vi "SaveExperimentInfo.vi"(10 "Filename":path, 11 "MeasureConfig":T1={"Bead locations"=[{"X"=0, "Y"=0}], "ROI"=0, "Experiment base path"=path "", "Image output subdir"="images", "Output mode"=enum."None", "Traces output subdir"="traces", "QTrk Settings"={"Image width"=150, "Image height"=150, "Number of threads (CPU based)"=-1, "CUDA Device"=200, "COM Background correction factor"=128.0, "ZLUT MinRadius"=32.0, "ZLUT Radial sample density"=2.0, "ZLUT Angular sample density"=5.0, "ZLUT ROI Coverage"=50.0, "QI Iterations"=64, "QI MinRadius"=2.0, "QI Radial sample density"=64.0, "QI Angular sample density"=64.0, "QI ROI Coverage"=2.0, "QI Angular Step \nIteration Factor"=30.0, "XCOR Profile Length"=0, "XCOR Profile Width"=2, "XCOR Iterations"=32, "Gaussian 2D Fit Iterations"=8, "Gaussian 2D Sigma (pixels)"=3.0, "Downsample"=0}, "Tracking Config"={"Number of steps"=150, "ZLUT stepsize (um)"=150.0, "Z correction factor"=-1.0, "Start piezo Z (um)"=200.0, "Pixel size (nm)"=128.0, "2D Localization Type"=enum."Quadrant Interpolation", "Z Command (None)"=enum."Nothing", "Z Piezo scale"=FALSE, "ZLUT Building\nimages per frame"=1, "ZLUT Bias correction planes"=1}, "Experiment Name"="", "Program"={"Commands"=[], "Motor Axis accuracy conditions"={"Magnet Z"=0.0, "Magnet rotation"=0.0, "Camera"={"X"=0.0, "Y"=0.0}, "Piezo XY"={"X"=0.0, "Y"=0.0}, "Piezo Z"=0.0}, "Axis flags"={"Magnet Z"=FALSE, "Magnet rotation"=FALSE, "Camera"={"X"=FALSE, "Y"=FALSE}, "Piezo XY"={"X"=FALSE, "Y"=FALSE}, "Piezo Z"=FALSE}}, "ZLUT"=[], "Camera settings"={"Framerate (Hz)"=60, "Exposure time (us)"=5000, "Image size"={"Width"=1280, "Height"=1024}, "Number of buffers"=30}, "Experiment Script"="", "Max frames in memory"=2, "Save traces as binary"=FALSE, "Pixel Calibration Gain Image"="camera_calib_gain.bin", "Pixel Calibration Offset Image"="camera_calib_gain.bin", "Use pixel calibration images"=FALSE, "Internal camera settings"="", "Trace write interval"=100, "ExperimentComment"=""} {"QTrk Settings"."QI ROI Coverage" format="%_2g"; "QTrk Settings"."QI MinRadius" format="%.2f"; "QTrk Settings"."QI Angular sample density" format="%.3f"; "QTrk Settings"."QI Radial sample density" format="%.2f"; "QTrk Settings"."ZLUT Radial sample density" format="%.2f"; "QTrk Settings"."ZLUT MinRadius" format="%.2f"}) -> ()   [LabVIEW 2011]
uses:
  Typedefs/MeasureConfigType.ctl
  Typedefs/MeasureConfigOutputMode.ctl
  qtrk/QTrkLVBinding/QTrkSettings.ctl
  Typedefs/TrackingConfigType.ctl
  qtrk/QTrkLVBinding/QTrkLocalizationType.ctl
  qtrk/QTrkLVBinding/QTrkZCommandType.ctl
  ExperimentProgram/ExperimentProgramType.ctl
  ExperimentProgram/ExProgCommandType.ctl
  ExperimentProgram/ExProgCommandEnumType.ctl
  Motors/MotorAxisEnum.ctl
  Motors/MotorPosType.ctl
  Typedefs/XYf.ctl
  Motors/MotorPosFlagsType.ctl
  Camera/GenericCameraConfigType.ctl
panel:
  # "(used for commands with string parameters)"
  # "-2: Use all devices\n-1: Use best device"
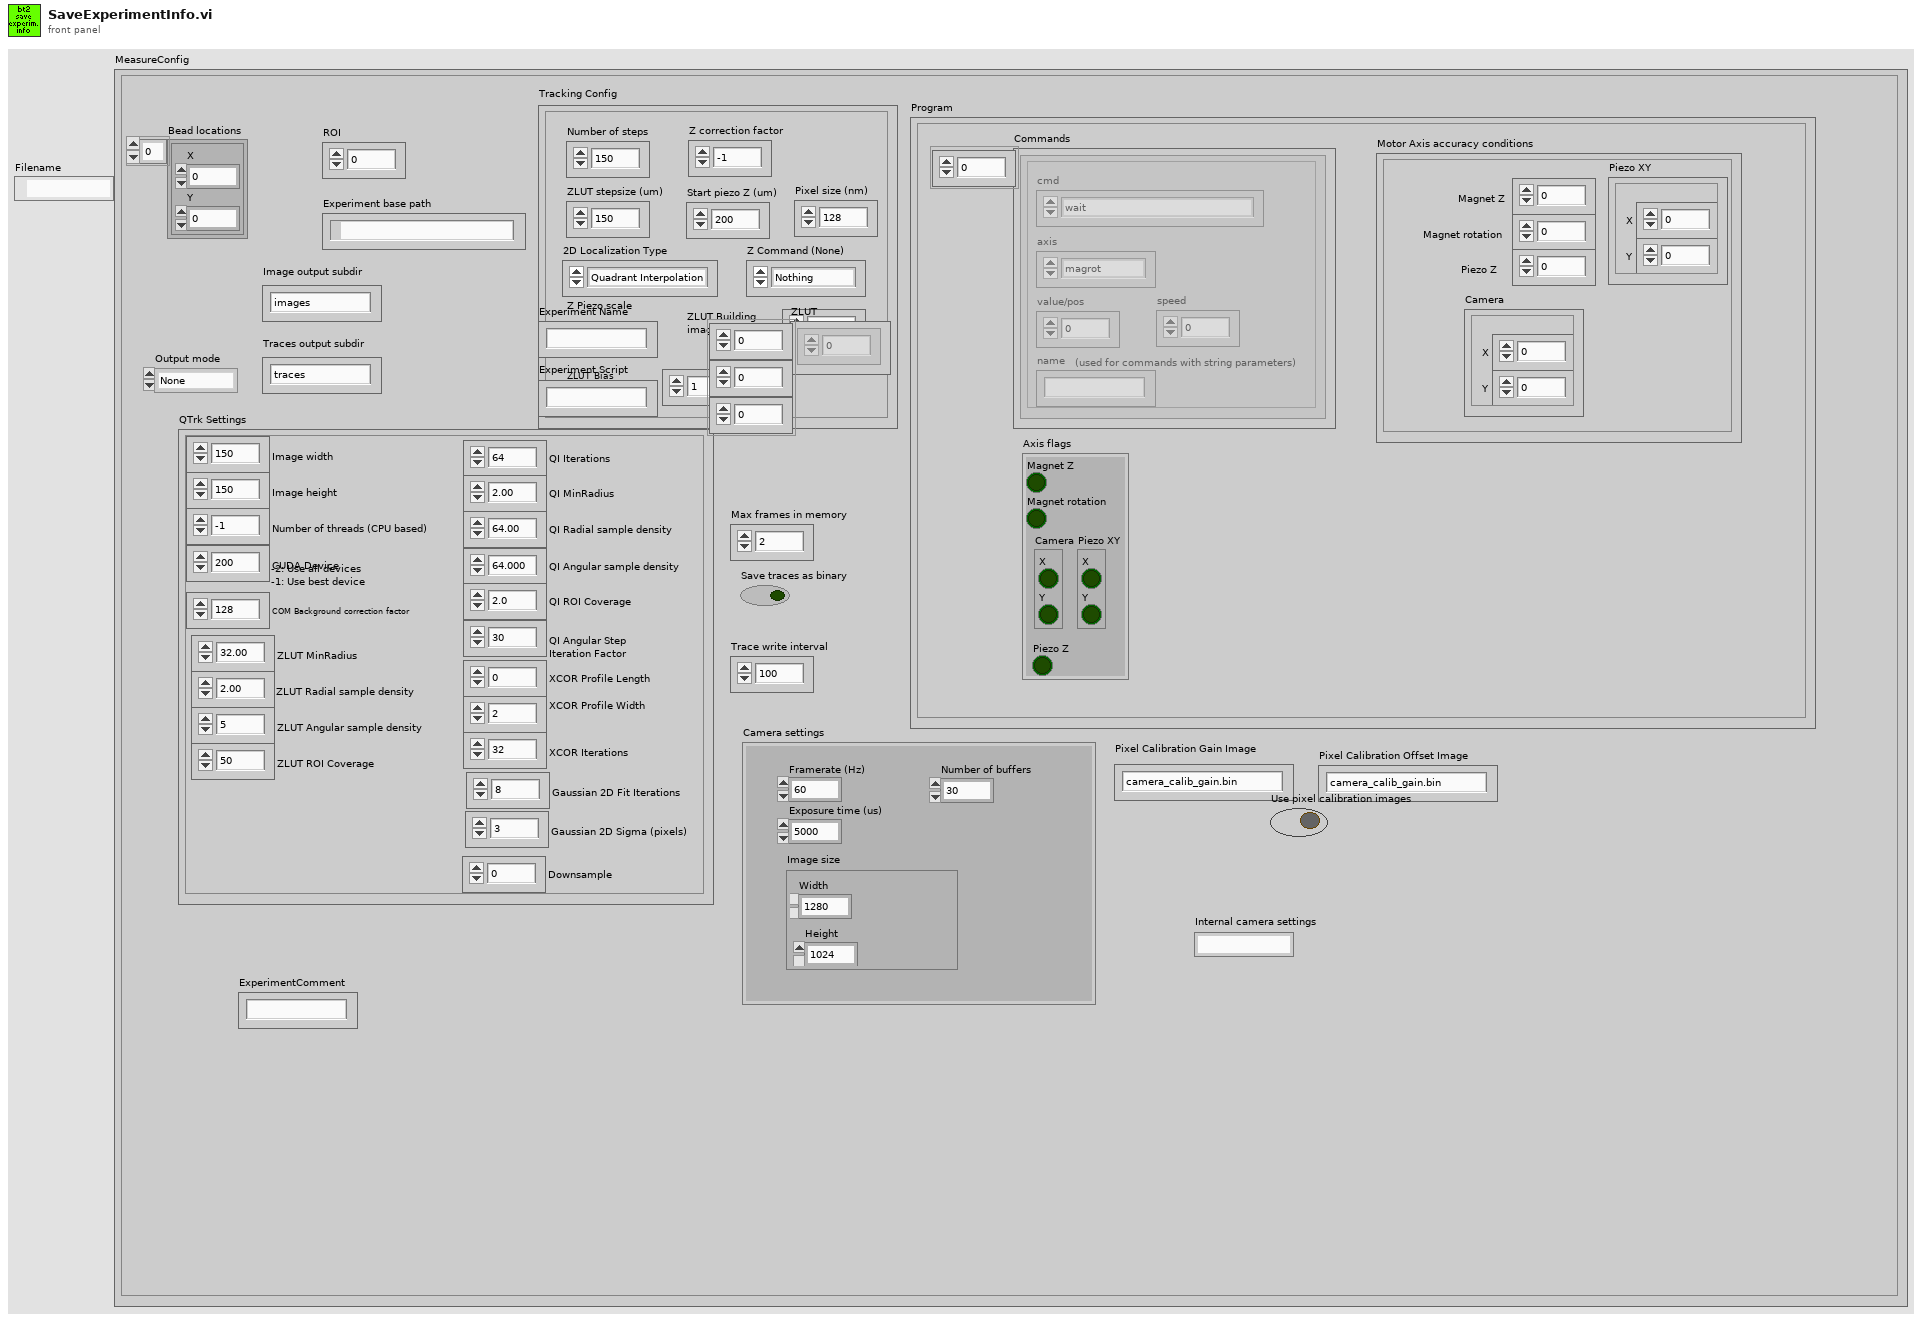
[diagram p1: front panel]
types:
  T1 = typedef "MeasureConfigType.ctl" = cluster{"Bead locations":cluster{"X":i32, "Y":i32}[], "ROI":i32, "Experiment base path":path, "Image output subdir":string, "Output mode":T2, "Traces output subdir":string, "QTrk Settings":T3, "Tracking Config":T4, "Experiment Name":string, "Program":T7, "ZLUT":sgl[][][], "Camera settings":T14, "Experiment Script":string, "Max frames in memory":i32, "Save traces as binary":bool, "Pixel Calibration Gain Image":string, "Pixel Calibration Offset Image":string, "Use pixel calibration images":bool, "Internal camera settings":string, "Trace write interval":i32, "ExperimentComment":string}
  T2 = typedef "MeasureConfigOutputMode.ctl" = enum16{"None", "Track", "SaveImages"}
  T3 = typedef "QTrkSettings.ctl" = cluster{"Image width":i32, "Image height":i32, "Number of threads (CPU based)":i32, "CUDA Device":i32, "COM Background correction factor":sgl, "ZLUT MinRadius":sgl, "ZLUT Radial sample density":sgl, "ZLUT Angular sample density":sgl, "ZLUT ROI Coverage":sgl, "QI Iterations":i32, "QI MinRadius":sgl, "QI Radial sample density":sgl, "QI Angular sample density":sgl, "QI ROI Coverage":sgl, "QI Angular Step \nIteration Factor":sgl, "XCOR Profile Length":i32, "XCOR Profile Width":i32, "XCOR Iterations":i32, "Gaussian 2D Fit Iterations":i32, "Gaussian 2D Sigma (pixels)":sgl, "Downsample":i32}
  T4 = typedef "TrackingConfigType.ctl" = cluster{"Number of steps":i32, "ZLUT stepsize (um)":sgl, "Z correction factor":sgl, "Start piezo Z (um)":sgl, "Pixel size (nm)":sgl, "2D Localization Type":T5, "Z Command (None)":T6, "Z Piezo scale":bool, "ZLUT Building\nimages per frame":i32, "ZLUT Bias correction planes":i32}
  T5 = typedef "QTrkLocalizationType.ctl" = enum16{"Center-of-Mass", "1D Cross-Correlation", "Quadrant Interpolation", "Gaussian 2D MLE", "QI + ZLUTAlign", "ZLUTAlign", "QI + FourierLUT"}
  T6 = typedef "QTrkZCommandType.ctl" = enum16{"Nothing", "ComputeZ", "BuildRadialZLUT", "BuildImageZLUT", "RadialZLUT+ImageZLUT"}
  T7 = typedef "ExperimentProgramType.ctl" = cluster{"Commands":T8[], "Motor Axis accuracy conditions":T11, "Axis flags":T13}
  T8 = typedef "ExProgCommandType.ctl" = cluster{"cmd":T9, "axis":T10, "value/pos":dbl, "speed":dbl, "name":string}
  T9 = typedef "ExProgCommandEnumType.ctl" = enum16{"wait", "move", "event", "idle", "when", "section", "stop"}
  T10 = typedef "MotorAxisEnum.ctl" = enum16{"no axis", "magrot", "magpos", "px", "py", "pz", "camx", "camy"}
  T11 = typedef "MotorPosType.ctl" = cluster{"Magnet Z":dbl, "Magnet rotation":dbl, "Camera":T12, "Piezo XY":T12, "Piezo Z":dbl}
  T12 = typedef "XYf.ctl" = cluster{"X":sgl, "Y":sgl}
  T13 = typedef "MotorPosFlagsType.ctl" = cluster{"Magnet Z":bool, "Magnet rotation":bool, "Camera":cluster{"X":bool, "Y":bool}, "Piezo XY":cluster{"X":bool, "Y":bool}, "Piezo Z":bool}
  T14 = typedef "GenericCameraConfigType.ctl" = cluster{"Framerate (Hz)":i32, "Exposure time (us)":i32, "Image size":cluster{"Width":i32, "Height":i32}, "Number of buffers":i32}
  T15 = enum16{"None", "Normalize", "NormalizeWithoutOffset"}
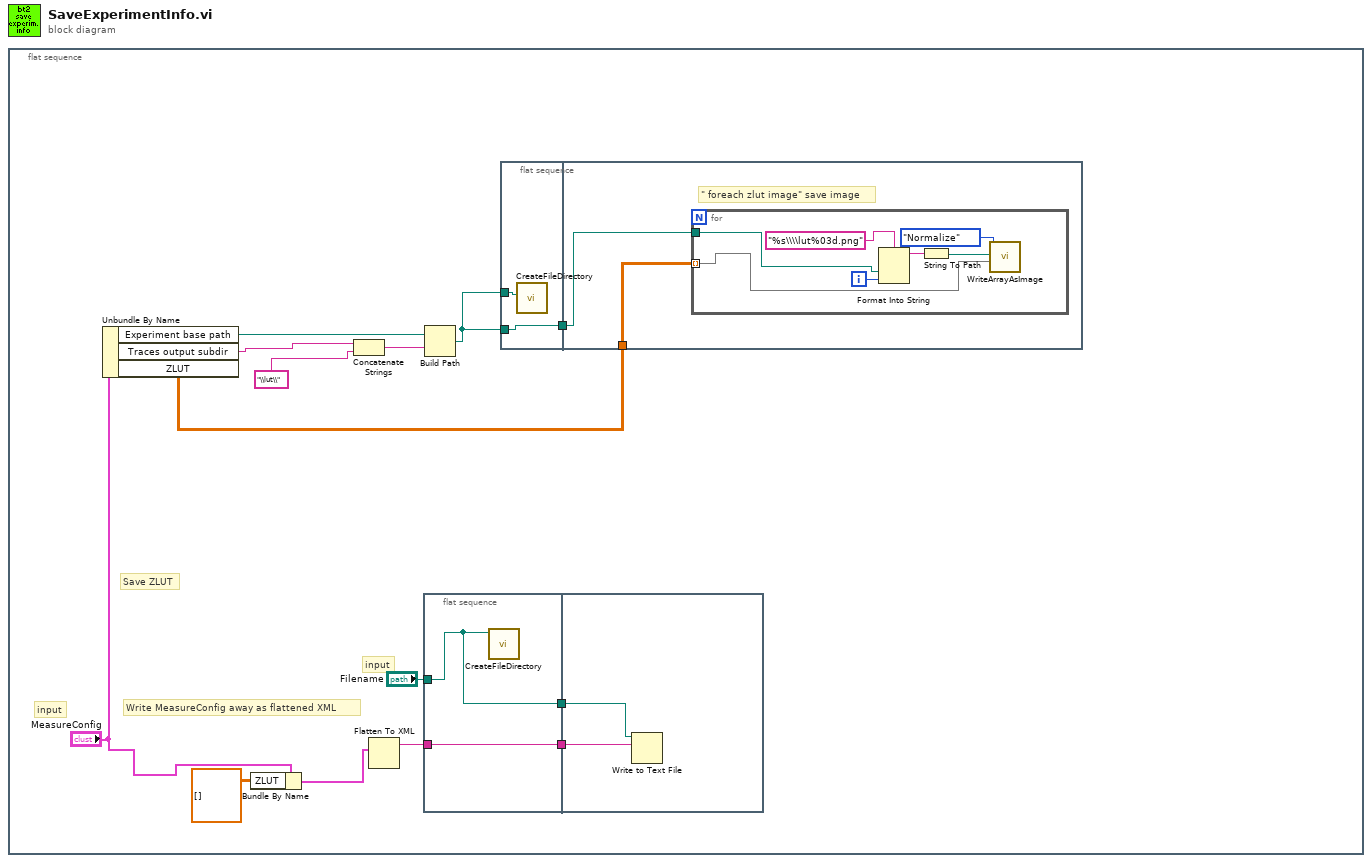
[diagram p0: block diagram]
diagram:
  n1 = flat-sequence {
    frame #0 {
      # "input"
      # "input"
      # "Write MeasureConfig away as flattened XML"
      # "Save ZLUT"
      n2 = Unbundle By Name("MeasureConfig") -> ("Experiment base path"=w12:path, "Traces output subdir"=w13:string, "ZLUT"=w1:sgl[][][])
      n3 = Bundle By Name(cluster="MeasureConfig", "ZLUT"=sgl[][][] []) -> (w5:T1)
      n4 = Concatenate Strings(w13, "\\lut\\" ("string")) -> (w11:string)
      n5 = Flatten To XML(anything=w5) -> (xml string=w9:string)
      n6 = flat-sequence {
        tunnel: "Filename" -> [w27]
        tunnel: w9 -> [w26]
        tunnel: [w27] -> w8
        tunnel: [w26] -> w7
        tunnel: w8 -> [w29]
        tunnel: w7 -> [w28]
        frame #0 {
          n7 = call "CreateFileDirectory.vi"("filename"=w27) -> ()  [unwired: 10 in, 1 out]
        }
        frame #1 {
          n8 = Write to Text File(file (use dialog)=w29, text=w28) -> ()  [unwired: 2 in, 3 out]
        }
      }
      n9 = Build Path(base path=w12, name or relative path=w11) -> (appended path=w3:path)
      n10 = flat-sequence {
        tunnel: w3 -> [w16]
        tunnel: w3 -> [w15]
        tunnel: [w15] -> w2
        tunnel: w2 -> [w18]
        tunnel: w1 -> [w17]
        frame #0 {
          n11 = call "CreateFileDirectory.vi"("directory"=w16) -> ()  [unwired: 10 in, 1 out]
        }
        frame #1 {
          # "\" foreach zlut image\" save image"
          n12 = for {
            tunnel: w17 -> [w20] mode=indexing
            tunnel: w18 -> [w19]
            i -> [w22]
            n13 = Format Into String(format string="%s\\\\lut%03d.png", w19, w22) -> (resulting string=w24:string)  [unwired: 2 in, 1 out]
            n14 = String To Path(string=w24) -> (path=w23:path)
            n15 = call "WriteArrayAsImage.vi"("Data"=w20, "File Path"=w23, "Normalize Mode"=T15."Normalize") -> ()  [unwired: 9 in]
          }
        }
      }
    }
  }
